vi "v1h_get_NC_string.vi"(3 "error in (no error)":errorcluster caption="错误输入（无错误）", 5 "refnum in":refnum<file>) -> (0 "error out":errorcluster, 1 "NC_string":string, 2 "refnum out":refnum<file>)   [LabVIEW 2016]
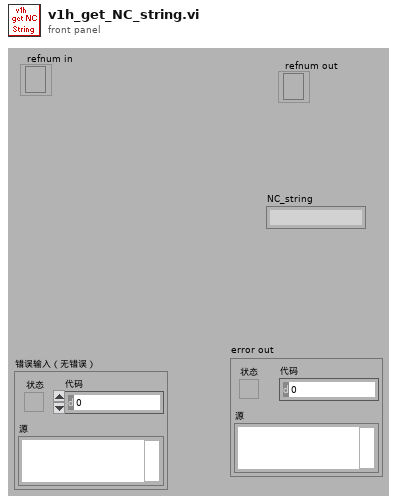
[diagram p1: front panel]
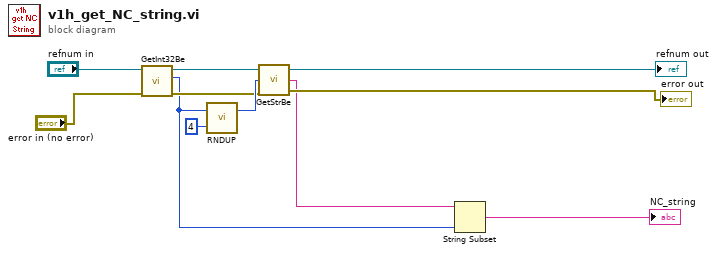
[diagram p0: block diagram]
diagram:
  n1 = call "GetInt32Be.vi"("error in (no error)"="error in (no error)", "refnum in"="refnum in") -> ("error out"=w8:errorcluster, "int32"=w3:i32, "refnum out"=w6:refnum<file>)  [unwired: 3 out]
  n2 = call "RNDUP.vi"("X_ALIGN"=4, "VAR"=w3) -> ("RUDUP"=w10:i32)  [unwired: 1 out]
  n3 = call "GetStrBe.vi"("error in"=w8, "nchars"=w10, "refnum in"=w6) -> ("error out"=→"error out":errorcluster, "str"=w4:string, "refnum out"=→"refnum out":refnum<file>)
  n4 = String Subset(string=w4, length (rest)=w3) -> (substring=→"NC_string":string)  [unwired: 1 out]
